vi "Teleop.vi"(10 "Match Info":T4={"Autonomous Elapsed Seconds"=0.0, "TeleOp Elapsed Seconds"=0.0, "Disabled Elapsed Seconds"=0.0, "Visited Autonomous"=FALSE, "Visited TeleOp"=FALSE, "Visited Disabled"=FALSE, "Autonomous Settings"={"Autonomous Style"=enum."Independent", "VI Refnum"=refnum}}, 11 "Call Context":T5) -> ()   [LabVIEW 2018]
doc: "This VI is called for each TeleOp packet received from the DS where the robot is not disabled. It is often used to read from the joysticks and update I/O or to update setpoints for timed control loops. It should complete and return within 20 milliseconds or it may miss DS packets."
uses:
  <vilib>/Rock Robotics/WPI/DriverStation/WPI_DriverStationDerivedRobotMode.ctl
  <vilib>/Rock Robotics/WPI/DriverStation/WPI_DriverStationMatch Info.ctl
  <vilib>/Rock Robotics/WPI/Solenoid/WPI_SolenoidValue.ctl
  <vilib>/Rock Robotics/WPI/ThirdParty/Phoenix-LabVIEW/Motor Controller/Controls/CTRE_Phoenix_MotorControl_ControlMode.ctl
  <vilib>/Rock Robotics/WPI/Utilities/WPI_GetSetVariantRefNum.vi
  <vilib>/Rock Robotics/WPI/Joystick/WPI_JoystickArcadeMapping.vi
  <vilib>/Rock Robotics/Network Tables/NT Write Boolean Array.vi
  <vilib>/Rock Robotics/Network Tables/NT Write Numeric Array.vi
  <vilib>/Rock Robotics/WPI/Solenoid/WPI_SolenoidSetEnum.vi
  <vilib>/Rock Robotics/WPI/ThirdParty/Phoenix-LabVIEW/Motor Controller/Get/CTRE_Phoenix_MotorController_GetSelectedSensorData.vi
  <vilib>/Rock Robotics/Network Tables/NT Read Boolean.vi
  Toolbox/Simple Limit Switch/Limits(Switch+Encoder).vi
  Toolbox/Simple Limit Switch/Limits(DoubleSwitch).vi
  Toolbox/Simple Limit Switch/Limits(SingleSwitch).vi
panel:
  out "Wrist Hold Pos":i32
  out "Elevator Out":dbl
  out "Elevator PID Out":dbl
  in  "Outer Invert Motor Limit":bool
  in  "Outer Invert Encoder Limit":bool=TRUE
  in  "Outer Limit":dbl format="%#_13g"
  in  "Horse Invert Encoder Limit":bool=TRUE
  in  "Wrist Invert Encoder Limit":bool
  in  "Elevator Invert Encoder Limit":bool=TRUE
  out "Horse Limit Switch":bool
  in  "Reset Horse Encoder":bool
  out "OuterStageSwitch":bool
  out "Wrist After Dangerzone":T1(ring)
  out "Elevator  After Dangerzone":T2(ring)
  in  "Elevator Auto":bool=TRUE
  in  "Elevator Output Range":cluster{"output high":dbl, "output low":dbl}={"output high"=0.2, "output low"=-0.75}
  in  "Elevator PID Gains":T3={"proportional gain (Kc)"=-1e-05, "integral time (Ti, min)"=0.0, "derivative time (Td, min)"=0.0}
  in  "Elevator Setpoints":dbl[](array[numeric])=[-10000.0, -10000.0, -10000.0, 267000.0, 237000.0, 440000.0]
  in  "Wrist Auto":bool=TRUE
  in  "Wrist Output Range":cluster{"output high":dbl, "output low":dbl}={"output high"=0.5, "output low"=-0.5}
  in  "Wrist PID Gains":T3={"proportional gain (Kc)"=2e-05, "integral time (Ti, min)"=0.0, "derivative time (Td, min)"=0.0}
  in  "Wrist Setpoints":dbl[](array[numeric])=[-7000.0, -7000.0, 80000.0, 70000.0, 136000.0, 45000.0, 29000.0, 65000.0, -65000.0]
  in  "Wrist Invert Motor Limit":bool
  out "Elevator Limit Switch Top":bool
  in  "Elevator Invert Motor Limit":bool=TRUE
  in  "Intake Encoder Limit":dbl=110000.0 format="%#_13g"
  in  "Intake Home Encoder Limit":dbl=-45000.0 format="%#_13g"
  in  "HorseDanger":i32=-600000
  in  "Horse  Encoder Limit":dbl=-190000.0 format="%#_13g"
  in  "Horse Invert Motor Limit":bool=TRUE
  out "Elevator Limit Switch":bool
  out "Elevator Encoder":i32=-47
  in  "Reset Elevator Encoder":bool
  out "Horse Encoder":i32
  in  "Reset Wrist Encoder":bool
  out "Intake Wrist Encoder":i32=4
  # "BETA POWER/DIRECTIONS\nElevator: Negative is up\nHorse: Negative is into robot\nOuter: Positive is down\nWrist: Negative is into robot"
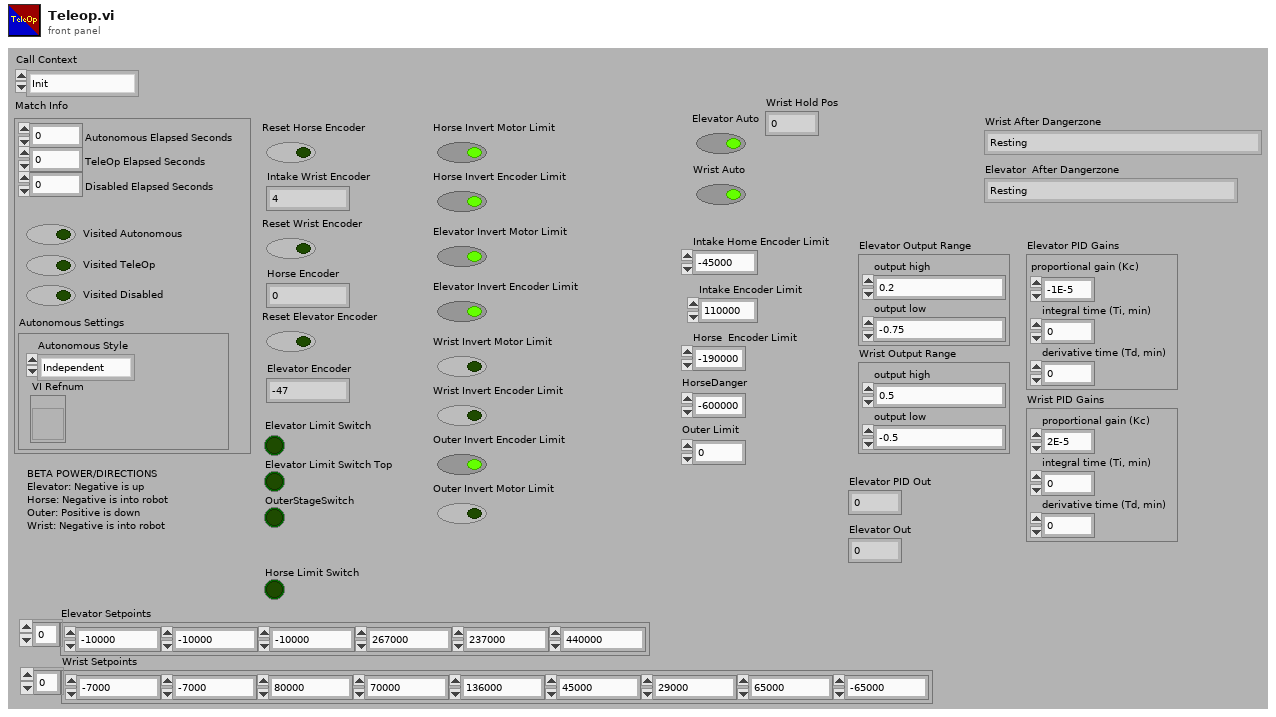
[diagram p1: front panel]
types:
  T1 = enum16{"Resting", "Hatch Ground Intake", "Hatch Place Low/Mid/CargoShip", "Hatch Place High", "Cargo Ground Intake", "Cargo Place Low/Mid", "Cargo Place High", "CargoShip Place Front", "CargoShip Place Back"}
  T2 = enum16{"Resting", "CargoShip Front", "CargoShip Back", "Cargo Mid", "Hatch Mid", "All High"}
  T3 = cluster{"proportional gain (Kc)":dbl, "integral time (Ti, min)":dbl, "derivative time (Td, min)":dbl}
  T4 = typedef "WPI_DriverStationMatch Info.ctl" = cluster{"Autonomous Elapsed Seconds":dbl, "TeleOp Elapsed Seconds":dbl, "Disabled Elapsed Seconds":dbl, "Visited Autonomous":bool, "Visited TeleOp":bool, "Visited Disabled":bool, "Autonomous Settings":cluster{"Autonomous Style":enum16{"Iterative", "Independent"}, "VI Refnum":refnum<vi>}}
  T5 = typedef "WPI_DriverStationDerivedRobotMode.ctl" = enum16{"Init", "Execute", "Stop"}
  T6 = typedef "WPI_SolenoidValue.ctl" = enum16{"Off", "On", "Forward", "Reverse"}
  T7 = enum16{"Intake Cargo", "Outtake Cargo", "Resting Cargo", "Reverse Cargo", "Intake Hatches", "Outtake Hatches", "Resting Hatches"}
  T8 = enum16{"Elevator Level 1", "Elevator Level 2", "Elevator Level 3"}
  T9 = typedef "CTRE_Phoenix_MotorControl_ControlMode.ctl" = u16
  T10 = cluster{"Intake Wheels Forwards":bool, "Elevator Shift":bool, "Intake Wheels Backwards":bool, "Drivetrain Shift":bool, "Elevator Outer Forwards":bool, "Elevator Outer Backwards":bool, "Hatch Telescope":bool, "Hatch Intake Clamp":bool, "Horse Drive Up":bool, "Horse Drive Down":bool, "Level 3 Climb":bool}
  T11 = typedef "WPI_JoystickDevRef.ctl" = cluster{"Device":T12}
  T12 = typedef "WPI_JoystickDeviceEnum.ctl" = enum16{"USB 0", "USB 1", "USB 2", "USB 3", "USB 4", "USB 5"}
  T13 = typedef "WPI_MotorControlDeviceRef.ctl" = cluster{"DeviceStatus":errorcluster, "Type":T14, "PWM":cluster{"PWM Channel":T15, "DeadBand":T16}, "CAN":cluster{"Device Number":u8, "SetOutput VI Ref":variant, "GetOutput VI Ref":variant, "Enable VI Ref":variant, "Disable VI Ref":variant, "Data":variant}, "Invert":bool, "DIO PWM":cluster{"PWM \"Enable\" Channel":T15, "DIOChannel":T17, "PWM Rate":dbl}}
  T14 = typedef "WPI_MotorControlType.ctl" = enum16{"PWM", "CAN", "DIO PWM"}
  T15 = typedef "FPGA_DIOPWMChannel.ctl" = enum8{"PWM 0", "PWM 1", "PWM 2", "PWM 3", "PWM 4", "PWM 5", "PWM 6", "PWM 7", "PWM 8", "PWM 9", "PWM MXP 0", "PWM MXP 1", "PWM MXP 2", "PWM MXP 3", "PWM MXP 4", "PWM MXP 5", "PWM MXP 6", "PWM MXP 7", "PWM MXP 8", "PWM MXP 9", "Invalid"}
  T16 = typedef "WPI_PWMDeadband.ctl" = cluster{"Name":string, "maxPositivePwm":i32, "minPositivePwm":i32, "centerPwm":i32, "maxNegativePwm":i32, "minNegativePwm":i32, "angularRange":u16}
  T17 = typedef "FPGA_DIOChannel.ctl" = enum8{"DIO 0", "DIO 1", "DIO 2", "DIO 3", "DIO 4", "DIO 5", "DIO 6", "DIO 7", "DIO 8", "DIO 9", "DIO MXP 0", "DIO MXP 1", "DIO MXP 2", "DIO MXP 3", "DIO MXP 4", "DIO MXP 5", "DIO MXP 6", "DIO MXP 7", "DIO MXP 8", "DIO MXP 9", "DIO MXP 10", "DIO MXP 11", "DIO MXP 12", "DIO MXP 13", "DIO MXP 14", "DIO MXP 15", "SPI Port CS1", "SPI Port CS2", "SPI Port CS3", "SPI Port MISO", "SPI Port MOSI", "Invalid"}
  T18 = typedef "WPI_SolenoidDevRef.ctl" = cluster{"DevStatus":errorcluster, "Pneumatics Control Module":u8, "Forward Solenoid Channel":T19, "Reverse Solenoid Channel":T19}
  T19 = typedef "WPI_SolenoidChannel.ctl" = enum8{"Solenoid 0", "Solenoid 1", "Solenoid 2", "Solenoid 3", "Solenoid 4", "Solenoid 5", "Solenoid 6", "Solenoid 7", "Invalid"}
  T20 = typedef "WPI_SwitchDevRef.ctl" = cluster{"DevStatus":errorcluster, "DIO Channel":T17, "CntIndex":T21, "Normally Closed":bool}
  T21 = typedef "FPGA_CounterCtrSystemIndex.ctl" = enum8{"Ctr 0", "Ctr 1", "Ctr 2", "Ctr 3", "Ctr 4", "Ctr 5", "Ctr 6", "Ctr 7", "Invalid"}
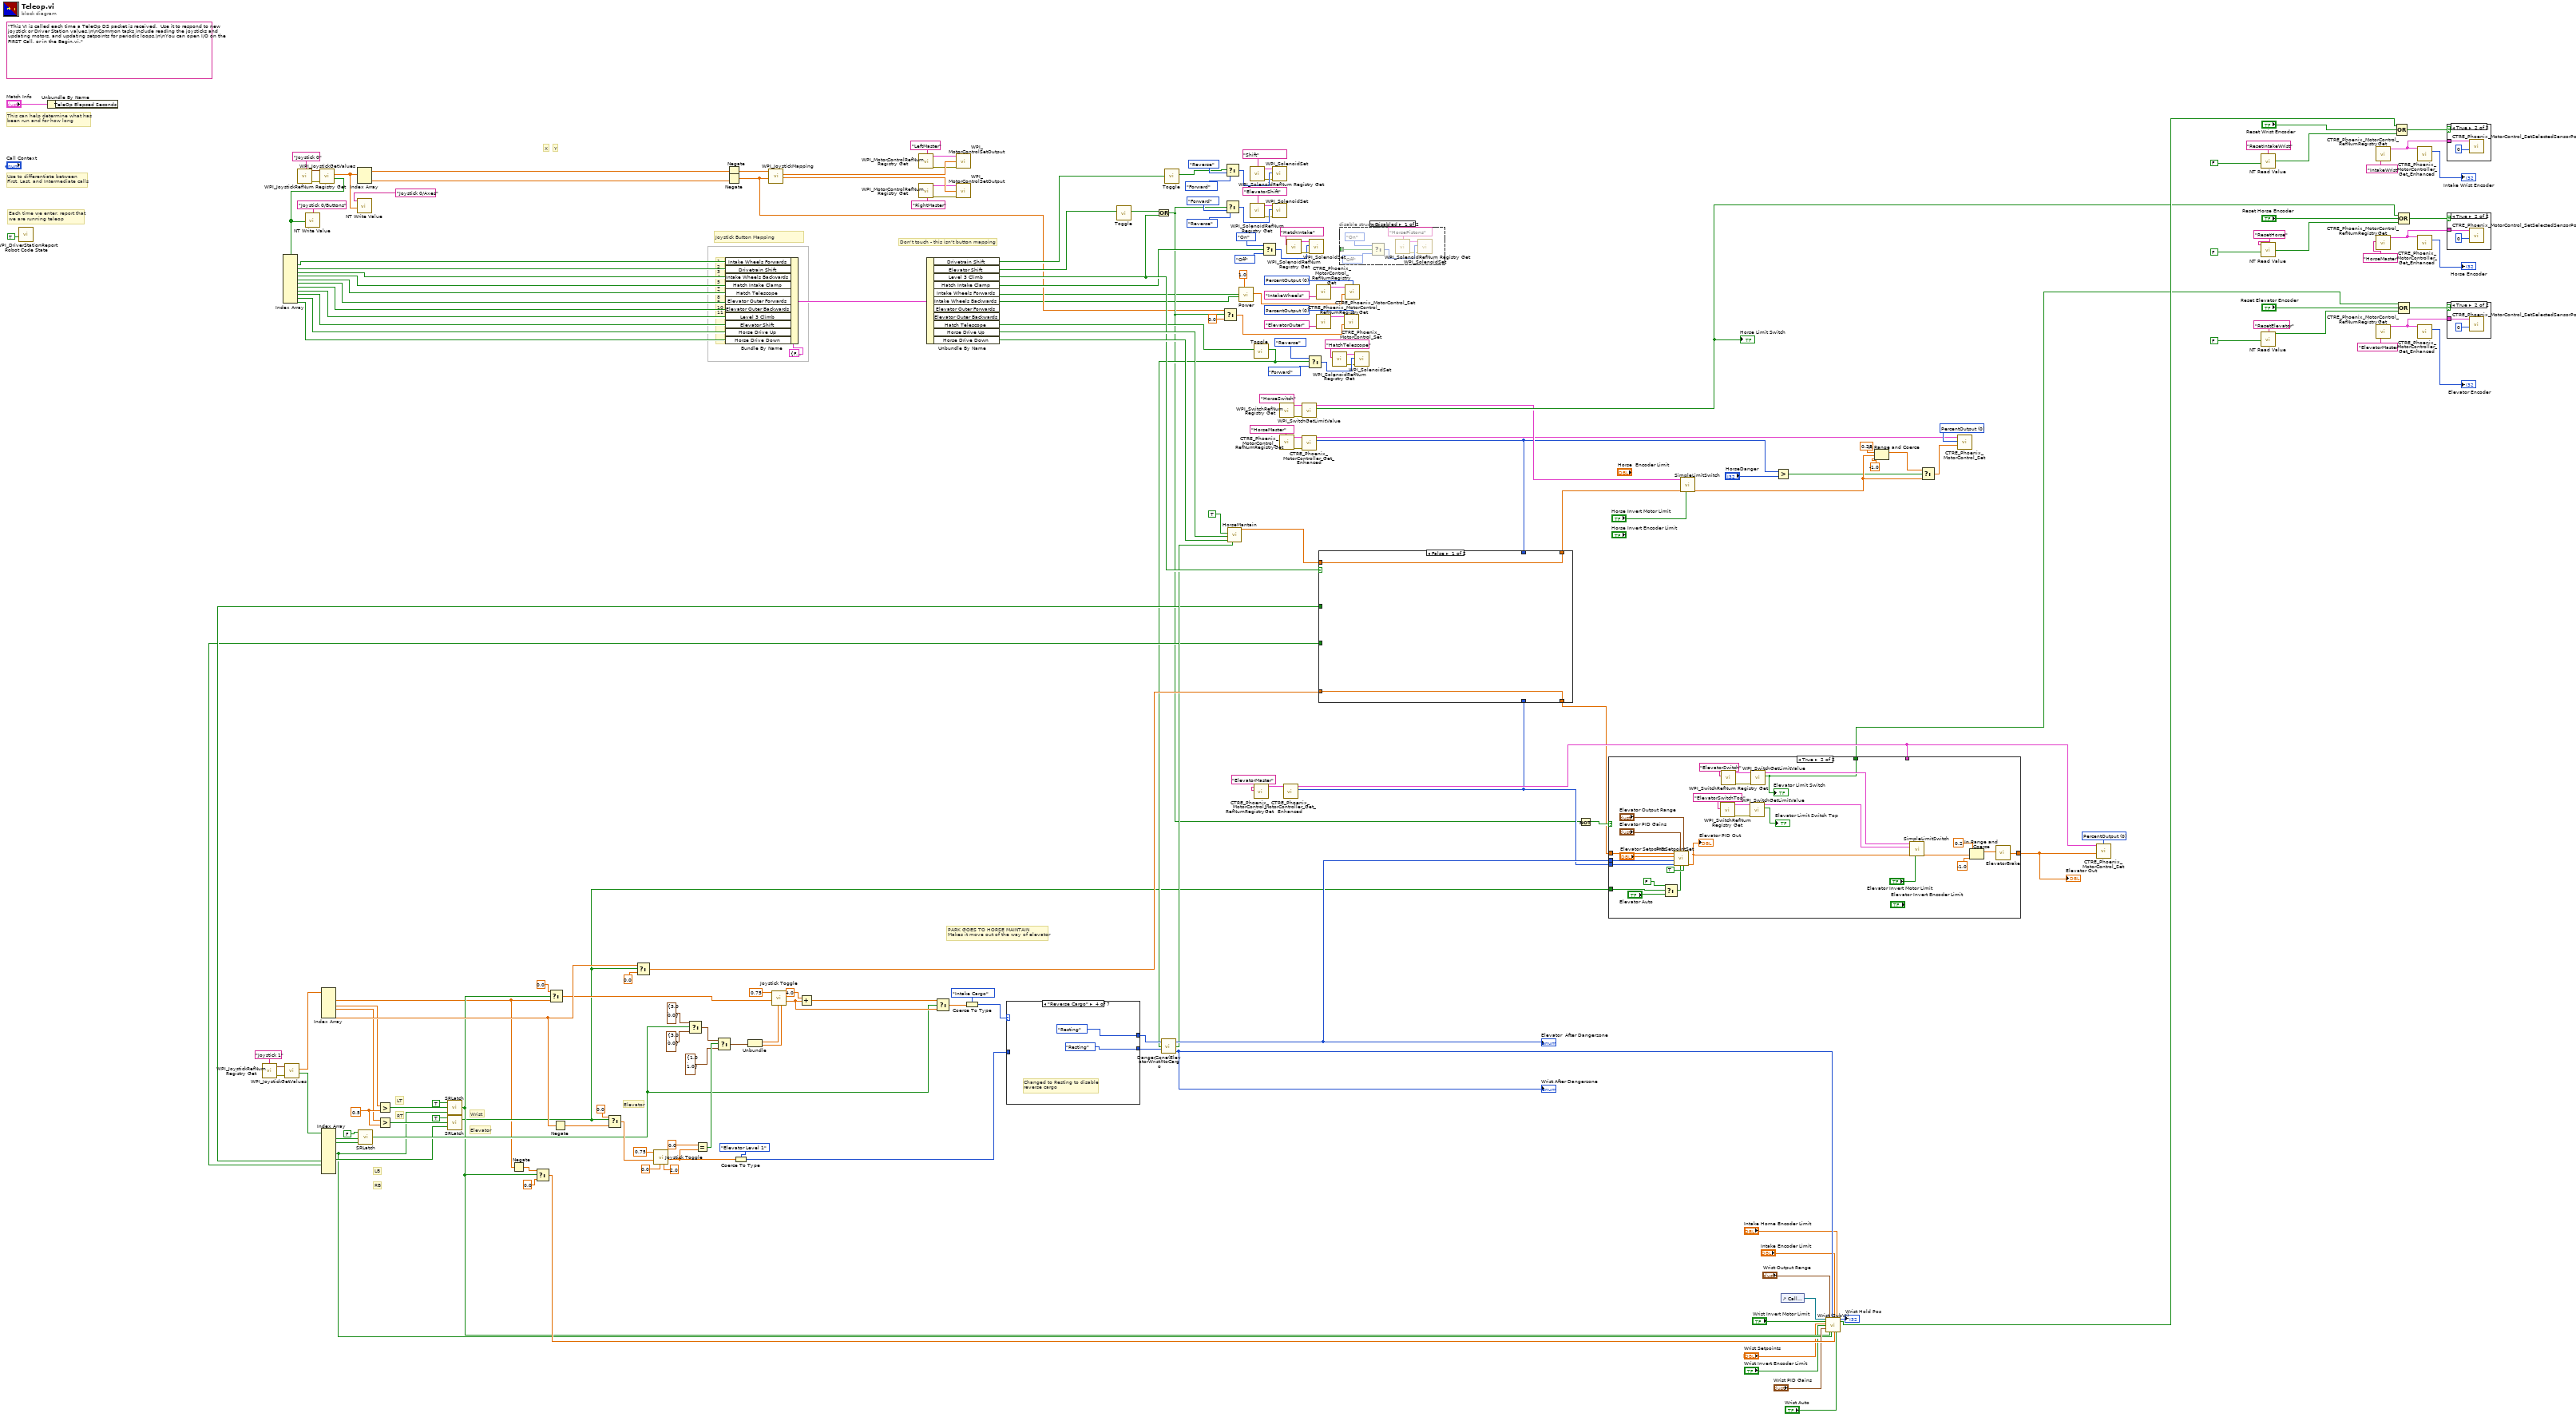
[diagram p0: block diagram]
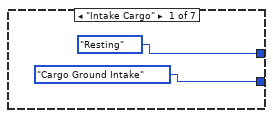
[diagram p3: hidden frame]
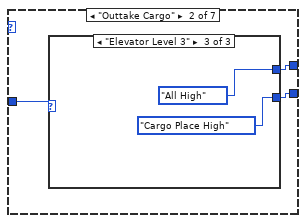
[diagram p4: hidden frame]
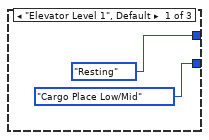
[diagram p5: hidden frame]
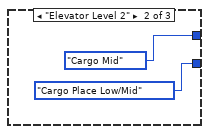
[diagram p6: hidden frame]
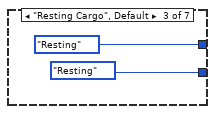
[diagram p7: hidden frame]
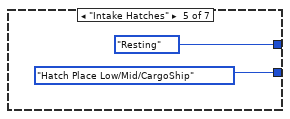
[diagram p8: hidden frame]
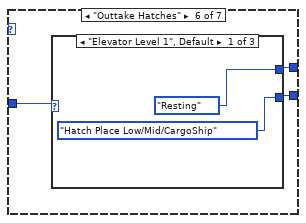
[diagram p9: hidden frame]
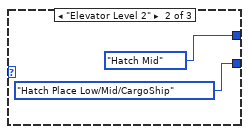
[diagram p10: hidden frame]
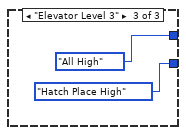
[diagram p11: hidden frame]
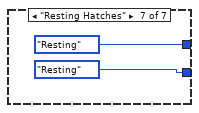
[diagram p12: hidden frame]
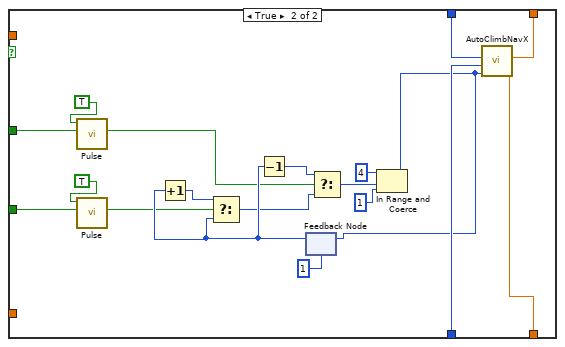
[diagram p13: hidden frame]
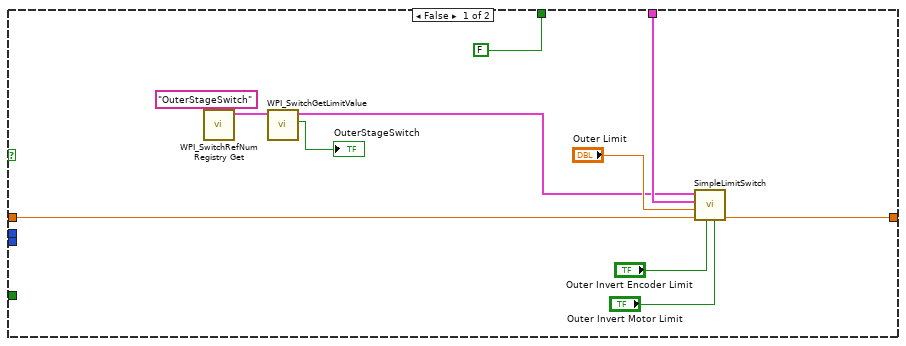
[diagram p14: hidden frame]
diagram:
  w32 = 0.5 ("t")
  w110 = T9 0 items=["PercentOutput"=0, "Position"=1, "Velocity"=2, "Current"=3, "Follower"=5, "MotionProfile"=6, "MotionMagic"=7, "MotionProfileArc"=10, "Disabled"=15] ("Control Mode")
  w114 = T9 0 items=["PercentOutput"=0, "Position"=1, "Velocity"=2, "Current"=3, "Follower"=5, "MotionProfile"=6, "MotionMagic"=7, "MotionProfileArc"=10, "Disabled"=15] ("Control Mode")
  w145 = T9 0 items=["PercentOutput"=0, "Position"=1, "Velocity"=2, "Current"=3, "Follower"=5, "MotionProfile"=6, "MotionMagic"=7, "MotionProfileArc"=10, "Disabled"=15] ("Control Mode")
  w147 = T9 0 items=["PercentOutput"=0, "Position"=1, "Velocity"=2, "Current"=3, "Follower"=5, "MotionProfile"=6, "MotionMagic"=7, "MotionProfileArc"=10, "Disabled"=15] ("Control Mode")
  (unwired) "This VI is called each time a TeleOp DS packet is received.  Use it to respond to new joystick or Driver Station values.\n\nCommon tasks include reading the joysticks and updating motors, and updating setpoints for periodic loops.\n\nYou can open I/O on the FIRST Call, or in the Begin.vi."
  # "Y"
  # "X"
  # "Elevator"
  # "Elevator"
  # "Wrist"
  # "LT"
  # "RT"
  # "RB"
  # "LB"
  # "Don't touch - this isn't button mapping"
  # "1\n2\n3\n4\n5\n6\n7\n8\n9\n10\n11"
  # "PARK GOES TO HORSE MAINTAIN\nMakes it move out of the way of elevator"
  # "Joystick Button Mapping"
  # "Each time we enter, report that\nwe are running teleop"
  # "Use to differentiate between\nFirst, Last, and Intermediate calls"
  # "This can help determine what has\nbeen run and for how long"
  n1 = call <vilib>:"WPI_DriverStationReport Robot Code State.vi"("TeleOp"=TRUE ("Autonomous")) -> ()  [unwired: 10 in, 1 out]
  n2 = Unbundle By Name("Match Info") -> ()  [unwired: 1 out]
  n3 = call <vilib>:"WPI_JoystickRefNum Registry Get.vi"("refnum name"="Joystick 1") -> ("error out"=w134:errorcluster, "JoystickDevRef"=w133:T11)  [unwired: 9 in]
  n4 = call <vilib>:"WPI_JoystickGetValues.vi"("error in (no error)"=w134, "JoystickDevRef"=w133) -> ("Buttons"=w121:bool[], "Axes"=w122:dbl[])  [unwired: 5 in, 3 out]
  n5 = call <vilib>:"WPI_JoystickRefNum Registry Get.vi"("refnum name"="Joystick 0") -> ("error out"=w175:errorcluster, "JoystickDevRef"=w206:T11)  [unwired: 1 in, 8 out]
  n6 = call <vilib>:"WPI_JoystickGetValues.vi"("error in (no error)"=w175, "JoystickDevRef"=w206) -> ("Buttons"=w172:bool[], "Axes"=w202:dbl[])  [unwired: 5 in, 3 out]
  n7 = Index Array(array=w172) -> (element #1=w190:bool, element #2=w200:bool, element #3=w199:bool, element #4=w198:bool, element #5=w197:bool, element #6=w196:bool, element #7=w195:bool, element #8=w194:bool, element #9=w193:bool, element #10=w192:bool, element #11=w191:bool)  [unwired: 11 in]
  n8 = call-poly <vilib>:"NT Write Value.vi"("Boolean Array"=w172, "Name"="Joystick 0/Buttons") -> ()  [unwired: 9 in, 1 out]
  n9 = Index Array(array=w122) -> (element #2=w12:dbl, element #3=w31:dbl, element #4=w30:dbl, element #6=w63:dbl)  [unwired: 6 in, 2 out]
  n10 = Index Array(array=w121) -> (element #1=w15:bool, element #4=w34:bool, element #5=w16:bool, element #6=w27:bool, element #7=w53:bool, element #8=w52:bool)  [unwired: 10 in, 4 out]
  n11 = Index Array(array=w202) -> (element #1=w151:dbl, element #2=w171:dbl)  [unwired: 2 in]
  n12 = call-poly <vilib>:"NT Write Value.vi"("Numeric Array"=w202, "Name"="Joystick 0/Axes") -> ()  [unwired: 9 in, 1 out]
  n13 = call "SRLatch.vi"("On"=w34, "Off"=w15, "Initial"=FALSE) -> ("Output"=w33:bool)
  n14 = Greater?(x=w31, y=w32) -> (0:w21:bool)
  n15 = Greater?(x=w30, y=w32) -> (0:w20:bool)
  n16 = call "SRLatch.vi"("On"=w16, "Off"=w21, "Initial"=TRUE) -> ("Output"=w14:bool)
  n17 = call "SRLatch.vi"("On"=w27, "Off"=w20, "Initial"=TRUE) -> ("Output"=w13:bool)
  n18 = Negate(x=w12) -> (-x=w65:dbl)
  n19 = Select(t=w65, s=w14, f=0.0) -> (s? t:f=w61:dbl)
  n20 = Select(t=0.0, s=w14, f=w12) -> (s? t:f=w57:dbl)
  n21 = Negate(x=w63) -> (-x=w56:dbl)
  n22 = Select(t=0.0, s=w13, f=w56) -> (s? t:f=w55:dbl)
  n23 = Select(t=w63, s=w13, f=0.0) -> (s? t:f=w62:dbl)
  n24 = call "Joystick Toggle.vi"("Max"=2.0, "Min"=0.0, "Value"=w55, "Range"=0.75) -> ("Output"=w83:dbl)  [unwired: 7 in]
  n25 = Select(t=cluster{"Range":dbl, "Range 2":dbl} {"Range"=3.0, "Range 2"=0.0}, s=w33, f=cluster{"Range":dbl, "Range 2":dbl} {"Range"=3.0, "Range 2"=0.0}) -> (s? t:f=w76:cluster{"Range":dbl, "Range 2":dbl})
  n26 = Equal?(x=0.0, y=w83) -> (x = y?=w75:bool)
  n27 = Select(t=w76, s=w75, f=cluster{"Range":dbl, "Range 2":dbl} {"Range"=1.0, "Range 2"=1.0}) -> (s? t:f=w77:cluster{"Range":dbl, "Range 2":dbl})
  n28 = Bundle By Name(cluster=T10 {"Intake Wheels Forwards"=FALSE, "Elevator Shift"=FALSE, "Intake Wheels Backwards"=FALSE, "Drivetrain Shift"=FALSE, "Elevator Outer Forwards"=FALSE, "Elevator Outer Backwards"=FALSE, "Hatch Telescope"=FALSE, "Hatch Intake Clamp"=FALSE, "Horse Drive Up"=FALSE, "Horse Drive Down"=FALSE, "Level 3 Climb"=FALSE} ("input cluster"), "Intake Wheels Forwards"=w190, "Drivetrain Shift"=w200, "Intake Wheels Backwards"=w199, "Hatch Intake Clamp"=w198, "Hatch Telescope"=w197, "Elevator Outer Forwards"=w196, "Elevator Outer Backwards"=w195, "Level 3 Climb"=w194, "Elevator Shift"=w193, "Horse Drive Up"=w192, "Horse Drive Down"=w191) -> (w189:T10)
  n29 = Negate(x=w151) -> (-x=w25:dbl)
  n30 = Negate(x=w171) -> (-x=w22:dbl)
  n31 = Coerce To Type(0:w83, 1:T8."Elevator Level 1") -> (2:w67:T8)
  n32 = Unbundle(w77) -> ("Range"=w79:dbl, "Range 2"=w78:dbl)
  n33 = call-poly <vilib>:"WPI_JoystickMapping.vi"("Y axis value"=w22, "X axis value"=w25) -> ("Right Motor Value"=w176:dbl, "Left Motor Value"=w177:dbl)  [unwired: 8 in]
  n34 = call "Joystick Toggle.vi"("Max"=w78, "Min"=w79, "Value"=w57, "Range"=0.75) -> ("Output"=w70:dbl)  [unwired: 7 in]
  n35 = Add(x=4.0 ("y"), y=w70) -> (x+y=w71:dbl)
  n36 = call <vilib>:"WPI_MotorControlRefNum Registry Get.vi"("refnum name"="LeftMaster") -> ("error out"=w131:errorcluster, "MotorControlDevRef"=w132:T13)  [unwired: 9 in]
  n37 = call <vilib>:"WPI_MotorControlRefNum Registry Get.vi"("refnum name"="RightMaster") -> ("error out"=w130:errorcluster, "MotorControlDevRef"=w129:T13)  [unwired: 9 in]
  n38 = Unbundle By Name(w189) -> ("Drivetrain Shift"=w170:bool, "Elevator Shift"=w90:bool, "Level 3 Climb"=w89:bool, "Hatch Intake Clamp"=w45:bool, "Intake Wheels Forwards"=w1:bool, "Intake Wheels Backwards"=w2:bool, "Hatch Telescope"=w43:bool, "Horse Drive Up"=w136:bool, "Horse Drive Down"=w137:bool)  [unwired: 2 out]
  n39 = Select(t=w71, s=w33, f=w70) -> (s? t:f=w73:dbl)
  n40 = call <vilib>:"WPI_MotorControlSetOutput.vi"("error in (no error)"=w131, "Output"=w177, "MotorControlDevRef"=w132) -> ()  [unwired: 6 in, 3 out]
  n41 = call <vilib>:"WPI_MotorControlSetOutput.vi"("error in (no error)"=w130, "Output"=w176, "MotorControlDevRef"=w129) -> ()  [unwired: 6 in, 3 out]
  n42 = Coerce To Type(0:w73, 1:T7."Intake Cargo") -> (2:w69:T7)
  n43 = case shown="\"Reverse Cargo\"" w69 {
    tunnel: [T1."Cargo Ground Intake" ("Wrist") w211 T1."Resting" ("Wrist") T1."Resting" ("Wrist") T1."Hatch Place Low/Mid/CargoShip" ("Wrist") w226 T1."Resting" ("Wrist")] -> w120
    tunnel: [T2."Resting" ("Elevator Level") w212 T2."Resting" ("Elevator Level") T2."Resting" ("Elevator Level") T2."Resting" ("Elevator Level") w227 T2."Resting" ("Elevator Level")] -> w118
    tunnel: w67 -> [_ w213 _ _ _ w228 _]
    frame "Intake Cargo" {
    }
    frame "Outtake Cargo" {
      n44 = case shown="\"Elevator Level 3\"" w213 {
        tunnel: [T2."Resting" ("Elevator Level") T2."Cargo Mid" ("Elevator Level") T2."All High" ("Elevator Level")] -> w212
        tunnel: [T1."Cargo Place Low/Mid" ("Wrist") T1."Cargo Place Low/Mid" ("Wrist") T1."Cargo Place High" ("Wrist")] -> w211
        frame "Elevator Level 1", Default {
        }
        frame "Elevator Level 2" {
        }
        frame "Elevator Level 3" {
        }
      }
    }
    frame "Resting Cargo", Default {
    }
    frame "Reverse Cargo" {
      # "Changed to Resting to disable\nreverse cargo"
    }
    frame "Intake Hatches" {
    }
    frame "Outtake Hatches" {
      n45 = case shown="\"Elevator Level 1\", Default" w228 {
        tunnel: [T2."Resting" ("Elevator Level") T2."Hatch Mid" ("Elevator Level") T2."All High" ("Elevator Level")] -> w227
        tunnel: [T1."Hatch Place Low/Mid/CargoShip" ("Wrist") T1."Hatch Place Low/Mid/CargoShip" ("Wrist") T1."Hatch Place High" ("Wrist")] -> w226
        frame "Elevator Level 1", Default {
        }
        frame "Elevator Level 2" {
        }
        frame "Elevator Level 3" {
        }
      }
    }
    frame "Resting Hatches" {
    }
  }
  n46 = call "Toggle.vi"("Input"=w90) -> ("Output"=w88:bool)  [unwired: 10 in]
  n47 = Or(x=w88, y=w89) -> (x .or. y?=w24:bool)
  n48 = call "Toggle.vi"("Input"=w170) -> ("Output"=w184:bool)  [unwired: 10 in]
  n49 = Select(t=w22, s=w24, f=0.0) -> (s? t:f=w26:dbl)
  n50 = Select(t=WPI_SolenoidValue."Reverse" ("Value"), s=w184, f=WPI_SolenoidValue."Forward" ("Value")) -> (s? t:f=w183:T6)
  n51 = Select(t=WPI_SolenoidValue."Forward" ("Value"), s=w24, f=WPI_SolenoidValue."Reverse" ("Value")) -> (s? t:f=w182:T6)
  n52 = call "Power.vi"("Positive Power"=1.0 ("Power"), "Negative"=w2, "Positive"=w1) -> ("Output"=w146:dbl)  [unwired: 8 in]
  n53 = call <vilib>:"WPI_SolenoidRefNum Registry Get.vi"("refnum name"="Shift") -> ("error out"=w173:errorcluster, "SolenoidDevRef"=w187:T18)  [unwired: 9 in]
  n54 = call <vilib>:"WPI_SolenoidRefNum Registry Get.vi"("refnum name"="ElevatorShift") -> ("error out"=w174:errorcluster, "SolenoidDevRef"=w179:T18)  [unwired: 9 in]
  n55 = call "Toggle.vi"("Input"=w43) -> ("Output"=w35:bool)  [unwired: 10 in]
  n56 = call "DangerZone(ElevatorWrist)NoCargo.vi"("Wrist"=w120, "Telescope Out"=w35, "Level"=w118) -> ("Wrist"=w135:T1, "Park Horse"=w59:bool, "Level"=w119:T2)
  "Elevator  After Dangerzone" <- w119
  "Wrist After Dangerzone" <- w135
  n57 = call "HorseMantain.vi"("Park"=w59, "Negative"=w137, "Positive"=w136, "HorseToggle"=TRUE) -> ("Power"=w95:dbl)  [unwired: 7 in]
  n58 = call <vilib>:"CTRE_Phoenix_MotorControl_RefNumRegistryGet.vi"("refnum name"="ElevatorMaster") -> ("PhoenixMotorControlDevRef"=w102:T13)  [unwired: 9 in, 1 out]
  n59 = Select(t=WPI_SolenoidValue."On" ("Value"), s=w45, f=WPI_SolenoidValue."Off" ("Value")) -> (s? t:f=w46:T6)
  n60 = call-poly <vilib>:"WPI_SolenoidSet.vi"("error in (no error)"=w173, "Value"=w183, "SolenoidDevRef"=w187) -> ()  [unwired: 7 in, 2 out]
  n61 = call-poly <vilib>:"WPI_SolenoidSet.vi"("error in (no error)"=w174, "Value"=w182, "SolenoidDevRef"=w179) -> ()  [unwired: 7 in, 2 out]
  n62 = call <vilib>:"WPI_SwitchRefNum Registry Get.vi"("refnum name"="HorseSwitch") -> ("error out"=w117:errorcluster, "SwitchDevRef"=w100:T20)  [unwired: 9 in]
  n63 = call <vilib>:"CTRE_Phoenix_MotorControl_RefNumRegistryGet.vi"("refnum name"="HorseMaster") -> ("error out"=w60:errorcluster, "PhoenixMotorControlDevRef"=w103:T13)  [unwired: 9 in]
  n64 = call-poly <vilib>:"CTRE_Phoenix_MotorController_Get_Enhanced.vi"("PhoenixMotorControlDevRef"=w102) -> ("PhoenixMotorControlDevRef"=w101:T13, "Position (Raw Sensor Units)"=w91:i32)  [unwired: 11 in, 2 out]
  n65 = call <vilib>:"WPI_SolenoidRefNum Registry Get.vi"("refnum name"="HatchIntake") -> ("error out"=w50:errorcluster, "SolenoidDevRef"=w49:T18)  [unwired: 9 in]
  n66 = call <vilib>:"WPI_SwitchGetLimitValue.vi"("error in (no error)"=w117, "SwitchDevRef"=w100) -> ("Switch Pressed"=w126:bool, "SwitchDevRef"=w99:T20)  [unwired: 7 in, 1 out]
  "Horse Limit Switch" <- w126
  n67 = call-poly <vilib>:"CTRE_Phoenix_MotorController_Get_Enhanced.vi"("PhoenixMotorControlDevRef"=w103, "error in"=w60) -> ("PhoenixMotorControlDevRef"=w36:T13, "Position (Raw Sensor Units)"=w96:i32)  [unwired: 10 in, 2 out]
  n68 = Select(t=WPI_SolenoidValue."Reverse" ("Value"), s=w35, f=WPI_SolenoidValue."Forward" ("Value")) -> (s? t:f=w41:T6)
  n69 = call-poly <vilib>:"WPI_SolenoidSet.vi"("error in (no error)"=w50, "Value"=w46, "SolenoidDevRef"=w49) -> ()  [unwired: 7 in, 2 out]
  n70 = call <vilib>:"CTRE_Phoenix_MotorControl_RefNumRegistryGet.vi"("refnum name"="IntakeWheels") -> ("PhoenixMotorControlDevRef"=w148:T13)  [unwired: 9 in, 1 out]
  n71 = call <vilib>:"CTRE_Phoenix_MotorControl_RefNumRegistryGet.vi"("refnum name"="ElevatorOuter") -> ("PhoenixMotorControlDevRef"=w144:T13)  [unwired: 9 in, 1 out]
  n72 = case shown="False" w89 {
    tunnel: w96 -> [_ w257]
    tunnel: [w237 w256] -> w94
    tunnel: [w238 w255] -> w92
    tunnel: w62 -> [w238 _]
    tunnel: w95 -> [w237 _]
    tunnel: w91 -> [_ w254]
    tunnel: w53 -> [_ w244]
    tunnel: w52 -> [_ w241]
    frame False {
    }
    frame True {
      n73 = call "Pulse.vi"("Input"=w244, "Rising Edge?"=TRUE) -> ("Output"=w250:bool)  [unwired: 9 in]
      n74 = call "Pulse.vi"("Input"=w241, "Rising Edge?"=TRUE) -> ("Output"=w247:bool)  [unwired: 9 in]
      n75 = feedback #1(1) -> (w252:i32)
      n76 = Increment(x=w252) -> (x+1=w248:i32)
      n77 = Select(t=w248, s=w247, f=w252) -> (s? t:f=w249:i32)
      n78 = Decrement(x=w252) -> (x-1=w251:i32)
      n79 = Select(t=w251, s=w250, f=w249) -> (s? t:f=w253:i32)
      n80 = In Range and Coerce(upper limit=4, x=w253, lower limit=1) -> (coerced(x)=w239:i32)  [unwired: 1 out]
      n81 = feedback-in #1(w239) -> ()
      n82 = call "AutoClimbNavX.vi"("Stage"=w239, "Elevator Encoder"=w254, "Horse Encoder"=w257) -> ("Elevator Output"=w255:dbl, "Horse Output"=w256:dbl)  [unwired: 7 in]
    }
  }
  n83 = call <vilib>:"WPI_SolenoidRefNum Registry Get.vi"("refnum name"="HatchTelescope") -> ("error out"=w37:errorcluster, "SolenoidDevRef"=w38:T18)  [unwired: 9 in]
  n84 = disable-structure shown="Disabled" {
    disable-tunnel: _ -> [w258 _]
    frame Disabled {
      n85 = Select(t=WPI_SolenoidValue."On" ("Value"), s=w258, f=WPI_SolenoidValue."Off" ("Value")) -> (s? t:f=w264:T6)
      n86 = call <vilib>:"WPI_SolenoidRefNum Registry Get.vi"("refnum name"="HorsePistons") -> ("error out"=w259:errorcluster, "SolenoidDevRef"=w261:T18)  [unwired: 9 in]
      n87 = call-poly <vilib>:"WPI_SolenoidSet.vi"("error in (no error)"=w259, "Value"=w264, "SolenoidDevRef"=w261) -> ()  [unwired: 7 in, 2 out]
    }
    frame Enabled {
    }
  }
  n88 = call <vilib>:"CTRE_Phoenix_MotorControl_Set.vi"("Output"=w26, "Control Mode"=w145, "PhoenixMotorControlDevRef"=w144) -> ()  [unwired: 7 in, 2 out]
  n89 = call <vilib>:"CTRE_Phoenix_MotorControl_Set.vi"("Output"=w146, "Control Mode"=w147, "PhoenixMotorControlDevRef"=w148) -> ()  [unwired: 7 in, 2 out]
  n90 = call-poly <vilib>:"WPI_SolenoidSet.vi"("error in (no error)"=w37, "Value"=w41, "SolenoidDevRef"=w38) -> ()  [unwired: 7 in, 2 out]
  n91 = Not(x=w24) -> (.not. x?=w98:bool)
  n92 = case shown="True" w98 {
    tunnel: w101 -> [w275 _]
    tunnel: w91 -> [_ w296]
    tunnel: w119 -> [_ w295]
    tunnel: w92 -> [w265 w292]
    tunnel: [w271 w290] -> w97
    tunnel: [FALSE ("Switch Pressed") w281] -> w93
    tunnel: w13 -> [_ w277]
    frame False {
      n93 = call <vilib>:"WPI_SwitchRefNum Registry Get.vi"("refnum name"="OuterStageSwitch") -> ("SwitchDevRef"=w270:T20)  [unwired: 9 in, 1 out]
      n94 = call <vilib>:"WPI_SwitchGetLimitValue.vi"("SwitchDevRef"=w270) -> ("Switch Pressed"=→"OuterStageSwitch":bool, "SwitchDevRef"=w267:T20)  [unwired: 8 in, 1 out]
      n95 = call-poly "SimpleLimitSwitch.vi"("Into Home Limit Is Pos (Encoder)"="Outer Invert Motor Limit", "Into Home Limit Is Pos (Motor)"="Outer Invert Encoder Limit", "Power In"=w265, "Encoder Limit"="Outer Limit", "Motor Ref"=w275, "Limit Switch Ref"=w267) -> ("Power Out"=w271:dbl)  [unwired: 5 in]
    }
    frame True {
      n96 = Select(t=FALSE ("Update"), s=w277, f="Elevator Auto") -> (s? t:f=w278:bool)
      n97 = call "PIDSetpointSet.vi"("Update"=TRUE, "Output Range"="Elevator Output Range", "Auto"=w278, "PID Gains"="Elevator PID Gains", "Encoder Position"=w296, "Level"=w295, "Setpoints"="Elevator Setpoints", "Manual Power"=w292) -> ("Power Out"=w294:dbl)  [unwired: 3 in]
      "Elevator PID Out" <- w294
      n98 = call <vilib>:"WPI_SwitchRefNum Registry Get.vi"("refnum name"="ElevatorSwitchTop") -> ("error out"=w283:errorcluster, "SwitchDevRef"=w285:T20)  [unwired: 9 in]
      n99 = call <vilib>:"WPI_SwitchRefNum Registry Get.vi"("refnum name"="ElevatorSwitch") -> ("error out"=w288:errorcluster, "SwitchDevRef"=w289:T20)  [unwired: 9 in]
      n100 = call <vilib>:"WPI_SwitchGetLimitValue.vi"("error in (no error)"=w283, "SwitchDevRef"=w285) -> ("Switch Pressed"=→"Elevator Limit Switch Top":bool, "SwitchDevRef"=w276:T20)  [unwired: 7 in, 1 out]
      n101 = call <vilib>:"WPI_SwitchGetLimitValue.vi"("error in (no error)"=w288, "SwitchDevRef"=w289) -> ("Switch Pressed"=w281:bool, "SwitchDevRef"=w286:T20)  [unwired: 7 in, 1 out]
      "Elevator Limit Switch" <- w281
      n102 = call-poly "SimpleLimitSwitch.vi"("Into Home Limit Is Pos"="Elevator Invert Motor Limit", "Power In"=w294, "2nd Limit Switch Ref"=w276, "Home Limit Switch Ref"=w286) -> ("Power Out"=w303:dbl)  [unwired: 7 in]
      n103 = In Range and Coerce(upper limit=0.2, x=w303, lower limit=-1.0) -> (coerced(x)=w291:dbl)  [unwired: 1 out]
      n104 = call "ElevatorBrake.vi"("Power In"=w291) -> ("Power Out"=w290:dbl)
    }
  }
  "Elevator Out" <- w97
  n105 = call-poly "SimpleLimitSwitch.vi"("Into Home Limit Is Pos (Motor)"="Horse Invert Motor Limit", "Power In"=w94, "Limit Switch Ref"=w99) -> ("Power Out"=w106:dbl)  [unwired: 8 in]
  n106 = Greater?(x=w96, y="HorseDanger") -> (0:w104:bool)
  n107 = control-ref of="Call Context"() -> (w7:refnum<vi>)
  n108 = call "Wrist (SubVI).vi"("Call Context"=w7, "Wrist Invert Motor Limit"="Wrist Invert Motor Limit", "Wrist Setpoints"="Wrist Setpoints", "Wrist Invert Encoder Limit"="Wrist Invert Encoder Limit", "Wrist PID Gains"="Wrist PID Gains", "Wrist Output Range"="Wrist Output Range", "Setpoint \nOverride"=w14, "Wrist Setpoint ID"=w135, "Safety Override"=w16, "Intake Encoder Limit"="Intake Encoder Limit", "Override Power"=w61, "Intake Home Encoder Limit"="Intake Home Encoder Limit", "Wrist Auto"="Wrist Auto") -> ("Wrist Hold Position"=→"Wrist Hold Pos":i32, "Switch Pressed"=w138:bool)  [unwired: 5 in]
  n109 = In Range and Coerce(upper limit=0.25, x=w106, lower limit=-1.0) -> (coerced(x)=w107:dbl)  [unwired: 1 out]
  n110 = Select(t=w107, s=w104, f=w106) -> (s? t:f=w105:dbl)
  n111 = call <vilib>:"CTRE_Phoenix_MotorControl_Set.vi"("Output"=w105, "Control Mode"=w114, "PhoenixMotorControlDevRef"=w36) -> ()  [unwired: 7 in, 2 out]
  n112 = call <vilib>:"CTRE_Phoenix_MotorControl_Set.vi"("Output"=w97, "Control Mode"=w110, "PhoenixMotorControlDevRef"=w101) -> ()  [unwired: 7 in, 2 out]
  n113 = call-poly <vilib>:"NT Read Value.vi"("Default Value"=FALSE, "Name"="ResetIntakeWrist") -> ("Boolean"=w159:bool)  [unwired: 8 in, 1 out]
  n114 = call-poly <vilib>:"NT Read Value.vi"("Default Value"=FALSE, "Name"="ResetHorse") -> ("Boolean"=w156:bool)  [unwired: 8 in, 1 out]
  n115 = call-poly <vilib>:"NT Read Value.vi"("Default Value"=FALSE, "Name"="ResetElevator") -> ("Boolean"=w141:bool)  [unwired: 8 in, 1 out]
  n116 = call <vilib>:"CTRE_Phoenix_MotorControl_RefNumRegistryGet.vi"("refnum name"="IntakeWrist") -> ("PhoenixMotorControlDevRef"=w167:T13)  [unwired: 9 in, 1 out]
  n117 = call <vilib>:"CTRE_Phoenix_MotorControl_RefNumRegistryGet.vi"("refnum name"="HorseMaster") -> ("PhoenixMotorControlDevRef"=w166:T13)  [unwired: 9 in, 1 out]
  n118 = call <vilib>:"CTRE_Phoenix_MotorControl_RefNumRegistryGet.vi"("refnum name"="ElevatorMaster") -> ("PhoenixMotorControlDevRef"=w161:T13)  [unwired: 9 in, 1 out]
  n119 = Compound Arithmetic op=OR(w138, "Reset Wrist Encoder", w159) -> (w123:bool)
  n120 = Compound Arithmetic op=OR(w126, "Reset Horse Encoder", w156) -> (w124:bool)
  n121 = Compound Arithmetic op=OR(w93, "Reset Elevator Encoder", w141) -> (w125:bool)
  n122 = call-poly <vilib>:"CTRE_Phoenix_MotorController_Get_Enhanced.vi"("PhoenixMotorControlDevRef"=w167) -> ("Position (Raw Sensor Units)"=→"Intake Wrist Encoder":i32)  [unwired: 11 in, 3 out]
  n123 = call-poly <vilib>:"CTRE_Phoenix_MotorController_Get_Enhanced.vi"("PhoenixMotorControlDevRef"=w166) -> ("Position (Raw Sensor Units)"=→"Horse Encoder":i32)  [unwired: 11 in, 3 out]
  n124 = call-poly <vilib>:"CTRE_Phoenix_MotorController_Get_Enhanced.vi"("PhoenixMotorControlDevRef"=w161) -> ("Position (Raw Sensor Units)"=→"Elevator Encoder":i32)  [unwired: 11 in, 3 out]
  n125 = case shown="True" w123 {
    tunnel: w167 -> [_ w305]
    frame False {
    }
    frame True {
      n126 = call <vilib>:"CTRE_Phoenix_MotorControl_SetSelectedSensorPosition.vi"("New Sensor Position"=0, "PhoenixMotorControlDevRef"=w305) -> ()  [unwired: 8 in, 2 out]
    }
  }
  n127 = case shown="True" w124 {
    tunnel: w166 -> [_ w307]
    frame False {
    }
    frame True {
      n128 = call <vilib>:"CTRE_Phoenix_MotorControl_SetSelectedSensorPosition.vi"("New Sensor Position"=0, "PhoenixMotorControlDevRef"=w307) -> ()  [unwired: 8 in, 2 out]
    }
  }
  n129 = case shown="True" w125 {
    tunnel: w161 -> [_ w309]
    frame False {
    }
    frame True {
      n130 = call <vilib>:"CTRE_Phoenix_MotorControl_SetSelectedSensorPosition.vi"("New Sensor Position"=0, "PhoenixMotorControlDevRef"=w309) -> ()  [unwired: 8 in, 2 out]
    }
  }
